vi "AFscanCoarseRange.vi"(6 "StopAfterMaxFrac":dbl=0.9 format="%#_13g", 7 "ScanRange":dbl=0.4, 8 "error in (no error)":errorcluster, 9 "ImageIn":T1, 10 "SessionIn":T2 caption="Session In", 11 "controller in":refnum<k24>) -> (0 "error out":errorcluster, 1 "Image Out":T1, 2 "Session Out":T2, 3 "controller out":refnum<k24>, 4 "MaxVal":dbl, 5 "BestZ":dbl)   [LabVIEW 2019]
uses:
  C:/Users/TTUHEP/Documents/LabVIEW/Other Models/2010/Bin/Aerotech.A3200.dll
  Other Models/2010/Bin/Aerotech.A3200.dll
  <vilib>/userDefined/High Color/IMAQdx.ctl
  <vilib>/vision/Image Controls.llb/IMAQ Image.ctl
  GlobalVariables.vi
  Other Models/2010/Motion/AbortSingle.vi
  <vilib>/vision/NI_Vision_Development_Module.lvlib
  <vilib>/vision/driver/NI_Vision_Acquisition_Software.lvlib
panel:
  out "XY Graph":T3(graph)
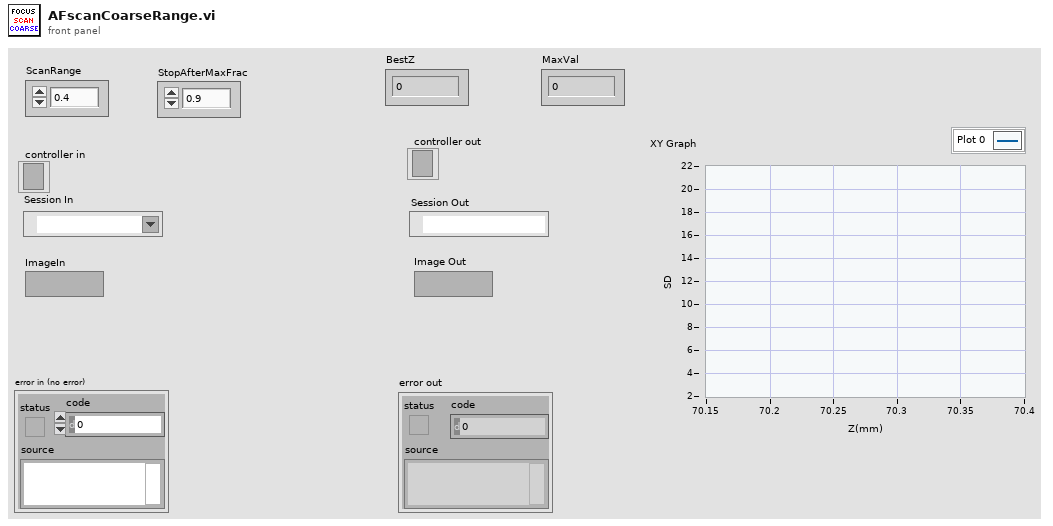
[diagram p1: front panel]
types:
  T1 = typedef "IMAQ Image.ctl" = refnum<image>
  T2 = typedef "IMAQdx.ctl" = refnum<k21>
  T3 = cluster{"Position Z":dbl, "Standard  Deviation":sgl}[]
  T4 = enum32{"Differentiation", "Gradient", "Prewitt", "Roberts", "Sigma", "Sobel"}
  T5 = typedef "Image Type" = u32
  T6 = cluster{"Position Z":dbl, "Standard  Deviation":sgl}
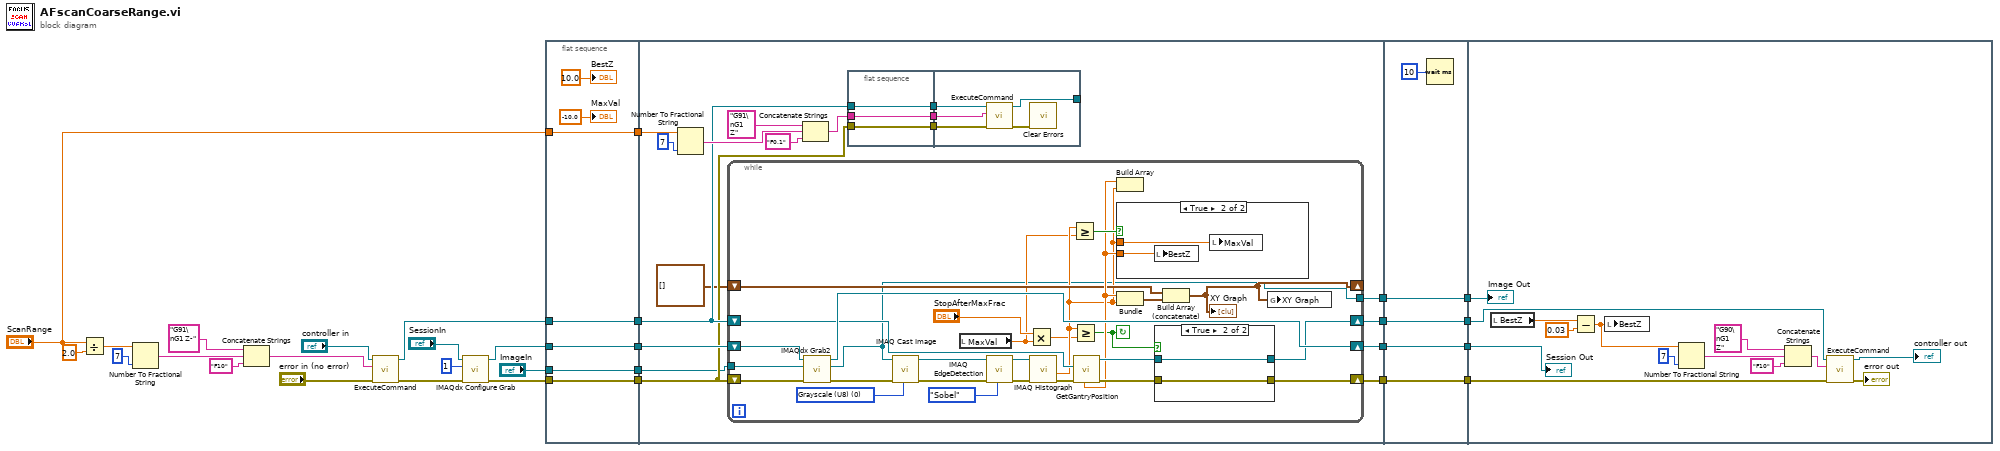
[diagram p0: block diagram]
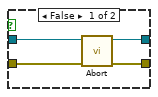
[diagram p2: hidden frame]
diagram:
  n1 = Divide(x="ScanRange", y=2.0) -> (x/y=w11:dbl)
  n2 = Number To Fractional String(number=w11, precision (6)=i16 7) -> (F-format string=w10:string)  [unwired: 2 in]
  n3 = Concatenate Strings("G91\nG1 Z-", w10, "F10" ("string")) -> (w9:string)
  n4 = call "ExecuteCommand.vi"("error in (no error)"="error in (no error)", "Command Code"=w9, "controller in"="controller in") -> ("error out"=w6:errorcluster, "controller out"=w18:refnum<k24>)  [unwired: 6 in, 1 out]
  n5 = call <vilib>:"IMAQdx Configure Grab.vi"("error in"=w6, "Number of Buffers"=u32 1, "Session In"="SessionIn") -> ("error out"=w5:errorcluster, "Session Out"=w17:T2)  [unwired: 7 in]
  n6 = flat-sequence {
    tunnel: w17 -> [w33]
    tunnel: w5 -> [w34]
    tunnel: "ImageIn" -> [w35]
    tunnel: "ScanRange" -> [w36]
    tunnel: w18 -> [w37]
    tunnel: [w37] -> w30
    tunnel: [w36] -> w29
    tunnel: [w35] -> w28
    tunnel: [w34] -> w27
    tunnel: [w33] -> w26
    tunnel: w30 -> [w46]
    tunnel: w29 -> [w55]
    tunnel: w28 -> [w38]
    tunnel: w27 -> [w45]
    tunnel: w26 -> [w52]
    tunnel: [w41] -> w25
    tunnel: [w54] -> w24
    tunnel: [w53] -> w23
    tunnel: [w39] -> w1
    tunnel: w25 -> [w104]
    tunnel: [w104] -> w22
    tunnel: w24 -> [w103]
    tunnel: [w103] -> w21
    tunnel: w23 -> [w102]
    tunnel: [w102] -> w20
    tunnel: [w100] -> w2
    tunnel: w1 -> [w100]
    tunnel: w22 -> [w118]
    tunnel: w21 -> [w108]
    tunnel: w20 -> [w112]
    tunnel: w2 -> [w106]
    frame #0 {
      "BestZ" <- 10.0 ("BestZ")
      "MaxVal" <- -10.0 ("MaxVal")
    }
    frame #1 {
      n7 = Number To Fractional String(number=w55, precision (6)=i16 7) -> (F-format string=w49:string)  [unwired: 2 in]
      n8 = while {
        tunnel: w38 -> [w83]
        shift-right: [w82] -> w54
        shift-left: w52 -> [w58]
        shift-right: [w69] -> w41
        shift-left: w46 -> [w75]
        shift-right: [w67] -> w53
        shift-left: w45 -> [w72]
        shift-right: [w63] -> _
        shift-left: T3 [] -> [w64]
        tunnel: [w56] -> w39
        stop <- w57 continue-if-true
        w79 = T5 0 items=["Grayscale (U8)", "Grayscale (I16)", "Grayscale (SGL)", "Complex (CSG)", "RGB (U32)", "HSL (U32)", "RGB (U64)", "Grayscale (U16)"] ("Image Type")
        n9 = call <vilib>:"IMAQdx Grab2.vi"("error in"=w72, "Image In"=w83, "Session In"=w58) -> ("error out"=w71:errorcluster, "Image Out"=w56:T1, "Session Out"=w82:T2)  [unwired: 5 in, 1 out]
        n10 = call "IMAQ Cast Image"("Image Type"=w79, "error in (no error)"=w71, "Image Src"=w56) -> ("error out"=w81:errorcluster, "Image Dst Out"=w80:T1)  [unwired: 7 in]
        n11 = local read "MaxVal"() -> (w60:dbl)
        n12 = call "IMAQ EdgeDetection"("Method"=T4."Sobel", "error in (no error)"=w81, "Image Src"=w80) -> ("error out"=w78:errorcluster, "Image Dst Out"=w77:T1)  [unwired: 7 in]
        n13 = Multiply(x="StopAfterMaxFrac", y=w60) -> (x*y=w59:dbl)
        n14 = call "IMAQ Histograph"("error in (no error)"=w78, "Image"=w77) -> ("error out"=w74:errorcluster, "Standard  Deviation"=w62:sgl)  [unwired: 6 in, 2 out]
        n15 = Greater Or Equal?(x=w62, y=w60) -> (x >= y?=w73:bool)
        n16 = Greater Or Equal?(x=w62, y=w59) -> (x >= y?=w57:bool)
        n17 = call "GetGantryPosition.vi"("error in (no error)"=w74, "Controller In"=w75) -> ("error out"=w68:errorcluster, "controller out"=w70:refnum<k24>, "Position Z"=w66:dbl)  [unwired: 3 in, 4 out]
        n18 = Build Array(w66, w62) -> ()  [unwired: 1 out]
        n19 = case shown="True" w73 {
          tunnel: w62 -> [_ w91]
          tunnel: w66 -> [_ w90]
          frame False {
          }
          frame True {
            n20 = local write "BestZ"(w90) -> ()
            n21 = local write "MaxVal"(w91) -> ()
          }
        }
        n22 = Bundle("Position Z"=w66, "Standard  Deviation"=w62) -> (w65:T6)  [unwired: 1 in]
        n23 = case shown="True" w57 {
          tunnel: w70 -> [w87 w89]
          tunnel: [w86 w89] -> w69
          tunnel: w68 -> [w85 w88]
          tunnel: [w84 w88] -> w67
          frame False {
            n24 = call-poly "Abort.vi"("error in (no error)"=w85, "controller in"=w87) -> ("error out"=w84:errorcluster, "controller out"=w86:refnum<k24>)  [unwired: 8 in]
          }
          frame True {
          }
        }
        n25 = Build Array (concatenate)(w64, w65) -> (w63:T3)
        "XY Graph" <- w63
        n26 = global write "GlobalVariables.vi" "XY Graph"(w63) -> ()
      }
      n27 = Concatenate Strings("G91\nG1 Z", w49, "F0.1" ("string")) -> (w48:string)
      n28 = flat-sequence {
        tunnel: w45 -> [w92]
        tunnel: w48 -> [w93]
        tunnel: w46 -> [w94]
        tunnel: [w94] -> w44
        tunnel: [w93] -> w43
        tunnel: [w92] -> w42
        tunnel: w44 -> [w99]
        tunnel: w43 -> [w98]
        tunnel: w42 -> [w97]
        tunnel: [w96] -> _
        frame #0 {
        }
        frame #1 {
          n29 = call "ExecuteCommand.vi"("error in (no error)"=w97, "Command Code"=w98, "controller in"=w99) -> ("error out"=w95:errorcluster, "controller out"=w96:refnum<k24>)  [unwired: 6 in, 1 out]
          n30 = call <vilib>:"Clear Errors.vi"("error in (no error)"=w95) -> ()  [unwired: 5 in, 2 out]
        }
      }
    }
    frame #2 {
      n31 = Wait (ms)(milliseconds to wait=u32 10) -> ()  [unwired: 1 out]
    }
    frame #3 {
      n32 = local read "BestZ"() -> (w111:dbl)
      n33 = Subtract(x=w111, y=0.03) -> (x-y=w109:dbl)
      n34 = local write "BestZ"(w109) -> ()
      n35 = Number To Fractional String(number=w109, precision (6)=i16 7) -> (F-format string=w114:string)  [unwired: 2 in]
      n36 = Concatenate Strings("G90\nG1 Z", w114, "F10" ("string")) -> (w113:string)
      n37 = call "ExecuteCommand.vi"("error in (no error)"=w112, "Command Code"=w113, "controller in"=w118) -> ("error out"=→"error out":errorcluster, "controller out"=→"controller out":refnum<k24>)  [unwired: 6 in, 1 out]
      "Session Out" <- w108
      "Image Out" <- w106
    }
  }
